vi "Check Status.vi"(8 "error in (no error)":errorcluster, 11 "Fluke Multimeter in":refnum<class "Fluke Multimeter.lvclass">) -> (0 "error out":errorcluster, 1 "Status":string, 2 "Ready?":bool, 3 "Fluke Multimeter out":refnum<class "Fluke Multimeter.lvclass">)   [LabVIEW 2009, in "Fluke Multimeter.lvclass"]
doc: "(Dynamic) Check if the instrument is powered on and update its member data with the instrument's current status. Optionally return a text status message."
uses:
  Fluke Multimeter.lvclass
  Utility Classes/Readable/Readable.lvclass
  Fluke Multimeter.lvclass/Fluke Multimeter.ctl
  Fluke 8840/Fluke 8840.lvlib
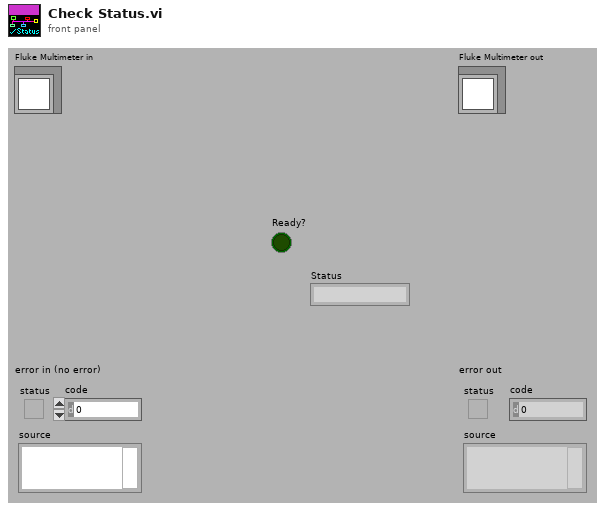
[diagram p1: front panel]
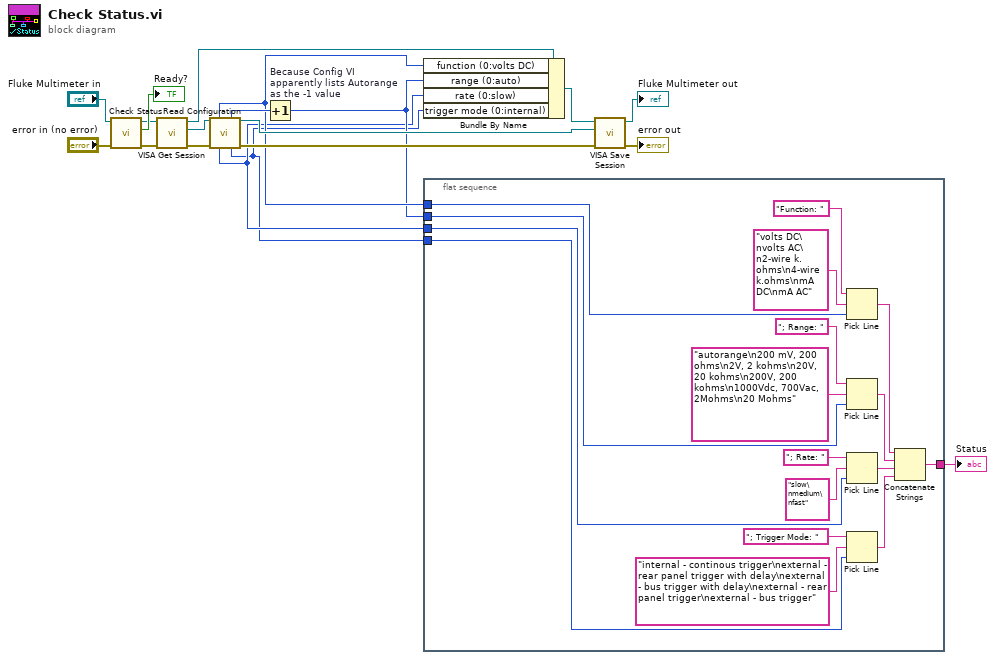
[diagram p0: block diagram]
diagram:
  n1 = call-parent "Check Status.vi"("error in (no error)"="error in (no error)", "Instrument in"="Fluke Multimeter in") -> ("error out"=w6:errorcluster, "Ready?"=→"Ready?":bool, "Instrument out"=w15:refnum<class "Fluke Multimeter.lvclass">)  [unwired: 7 out]
  n2 = call-dynamic "VISA Get Session.vi"("error in (no error)"=w6, "Instrument.lvclass in"=w15) -> ("error out"=w5:errorcluster, "VISA Resource Name"=w9:refnum<visa-resource-name>, "Instrument.lvclass out"=w12:refnum<class "Fluke Multimeter.lvclass">)  [unwired: 7 out]
  n3 = call "Read Configuration.vi"("VISA resource name"=w9, "error in (no error)"=w5) -> ("function"=w4:i32, "range"=w10:i32, "VISA resource name out"=w7:refnum<visa-resource-name>, "rate"=w2:i32, "trigger mode"=w1:i32, "error out"=w8:errorcluster)  [unwired: 8 out]
  n4 = Increment "Because Config VI\napparently lists Autorange\nas the -1 value"(x=w10) -> (x+1=w3:i32)
  n5 = Bundle By Name(cluster=w12, "function (0:volts DC)"=w4, "range (0:auto)"=w3, "rate (0:slow)"=w2, "trigger mode (0:internal)"=w1) -> (w11:refnum<class "Fluke Multimeter.lvclass">)
  n6 = flat-sequence {
    tunnel: [w34] -> w16
    tunnel: w4 -> [w32]
    tunnel: w3 -> [w29]
    tunnel: w2 -> [w24]
    tunnel: w1 -> [w23]
    frame #0 {
      n7 = Pick Line(string ("")="Function: ", multi-line string="volts DC\nvolts AC\n2-wire k.ohms\n4-wire k.ohms\nmA DC\nmA AC", line index=w32) -> (output string=w35:string)
      n8 = Pick Line(string ("")="; Range: ", multi-line string="autorange\n200 mV, 200 ohms\n2V, 2 kohms\n20V, 20 kohms\n200V, 200 kohms\n1000Vdc, 700Vac, 2Mohms\n20 Mohms", line index=w29) -> (output string=w28:string)
      n9 = Pick Line(string ("")="; Rate: ", multi-line string="slow\nmedium\nfast", line index=w24) -> (output string=w21:string)
      n10 = Pick Line(string ("")="; Trigger Mode: ", multi-line string="internal - continous trigger\nexternal - rear panel trigger with delay\nexternal - bus trigger with delay\nexternal - rear panel trigger\nexternal - bus trigger", line index=w23) -> (output string=w20:string)
      n11 = Concatenate Strings(w35, w28, w21, w20) -> (w34:string)
    }
  }
  n12 = call-dynamic "VISA Save Session.vi"("error in (no error)"=w8, "VISA Resource Name"=w7, "Instrument.lvclass in"=w11) -> ("error out"=→"error out":errorcluster, "Instrument.lvclass out"=→"Fluke Multimeter out":refnum<class "Fluke Multimeter.lvclass">)  [unwired: 7 out]
  "Status" <- w16
